vi "FA_ApplyRTEXEiniKeys.vi"(8 "Error In":errorcluster, 10 "Value In":string, 11 "INI Key Type":enum16{"Filename", "LaunchAppAtBoot"}(ring)) -> (0 "Error Out":errorcluster)   [LabVIEW 2014, in "FA_ApplyRTEXE.lvlib"]
uses:
  FA_ApplyRTEXE.lvlib
  FA_LocalStore API/source/VI Source/FA_LSCollections.ctl
  FA_LocalStore API/source/VI Source/FA_LSSpecialTypes.ctl
  <vilib>/Utility/config.llb/Write Key (Path).vi
  <vilib>/Utility/config.llb/Write Key (Boolean).vi
  <vilib>/Utility/config.llb/NI_LVConfig.lvlib
  FA_LocalStore API/source/VI Source/FA_LocalStore.lvlib
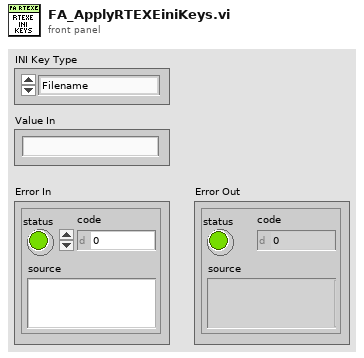
[diagram p1: front panel]
types:
  T1 = typedef "NI_LVConfig.lvlib/Config Data RefNum.ctl" = refnum<k1>
  T2 = typedef "FA_LocalStore.lvlib/FA_LSSpecialTypes.ctl" = string
  T3 = typedef "FA_LocalStore.lvlib/FA_LSCollections.ctl" = enum16{"Config", "ConfigItem", "FA_eTag", "FA_PlugIn"}
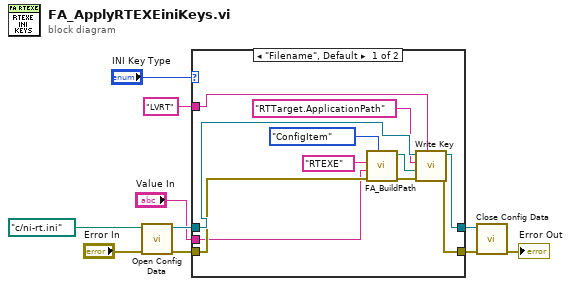
[diagram p0: block diagram]
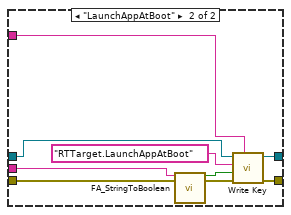
[diagram p2: hidden frame]
diagram:
  n1 = call <vilib>:"Open Config Data.vi"("error in (no error)"="Error In", "configuration file path"=path "c:/ni-rt.ini" ("appended path")) -> ("error out"=w8:errorcluster, "refnum"=w9:T1)  [unwired: 7 in, 1 out]
  n2 = case shown="\"Filename\", Default" "INI Key Type" {
    tunnel: w9 -> [w19 w29]
    tunnel: w8 -> [w13 w23]
    tunnel: [w20 w28] -> w7
    tunnel: [w21 w27] -> w6
    tunnel: "LVRT" ("section") -> [w17 w26]
    tunnel: "Value In" -> [w11 w25]
    frame "Filename", Default {
      n3 = call "FA_BuildPath.vi"("LSCollections"=FA_LSCollections."ConfigItem", "error in (no error)"=w13, "Item Name"=w11, "Special Type"=T2 "RTEXE") -> ("error out"=w12:errorcluster, "file path"=w14:path)  [unwired: 5 in, 1 out]
      n4 = call-poly <vilib>:"Write Key.vi"("section"=w17, "error in (no error)"=w12, "value"=w14, "key"="RTTarget.ApplicationPath", "refnum"=w19) -> ("error out"=w21:errorcluster, "refnum out"=w20:T1)  [unwired: 4 in, 1 out]
    }
    frame "LaunchAppAtBoot" {
      n5 = call "FA_StringToBoolean.vi"("Input String"=w25, "Error In"=w23) -> ("Boolean"=w24:bool, "Error Out"=w22:errorcluster)  [unwired: 16 in]
      n6 = call-poly <vilib>:"Write Key.vi"("section"=w26, "error in (no error)"=w22, "value"=w24, "key"="RTTarget.LaunchAppAtBoot", "refnum"=w29) -> ("error out"=w27:errorcluster, "refnum out"=w28:T1)  [unwired: 4 in, 1 out]
    }
  }
  n7 = call <vilib>:"Close Config Data.vi"("error in (no error)"=w6, "refnum"=w7) -> ("error out"=→"Error Out":errorcluster)  [unwired: 8 in, 1 out]
